vi "CmdString.vi"(8 "error in (no error)":errorcluster, 10 "String":string, 11 "VISA resource name":refnum<visa-resource-name>) -> (0 "error out":errorcluster, 2 "String out":string, 3 "VISA resource name out":refnum<visa-resource-name>)   [LabVIEW 2011]
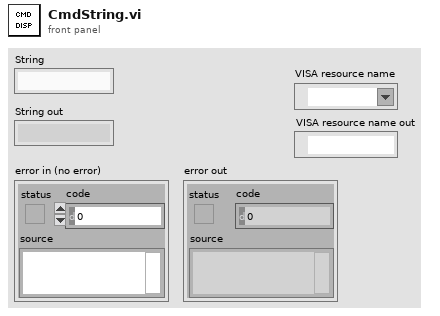
[diagram p1: front panel]
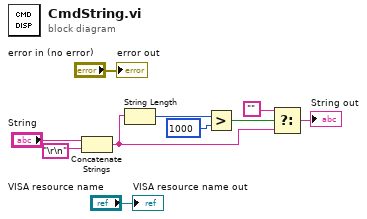
[diagram p0: block diagram]
diagram:
  n1 = Concatenate Strings("String", "\r\n") -> (w6:string)
  n2 = String Length(string=w6) -> (length=w4:i32)
  n3 = Greater?(x=w4, y=1000) -> (0:w2:bool)
  n4 = Select(t="", s=w2, f=w6) -> (s? t:f=→"String out":string)
  "error out" <- "error in (no error)"
  "VISA resource name out" <- "VISA resource name"
